vi "Write Listbox Data.vi"(8 "error in":errorcluster, 10 "Value":string[](array[string]), 11 "Listbox Ref in":refnum<vi>) -> (0 "error out":errorcluster, 3 "Listbox Ref out":refnum<vi>)   [LabVIEW 2020, in "G-Unicode.lvlib"]
uses:
  G-Unicode.lvlib
  Unicode/Controls/String Encoding.ctl
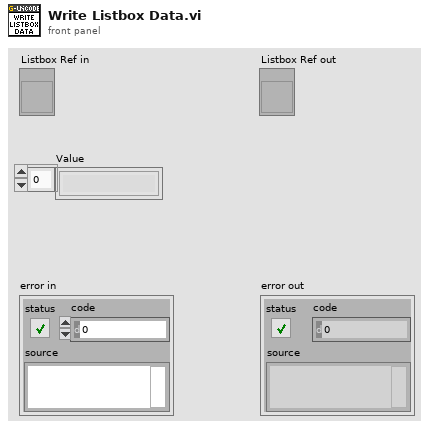
[diagram p1: front panel]
types:
  T1 = typedef "G-Unicode.lvlib/String Encoding.ctl" = enum16{"ANSI", "UTF-8", "UTF-16LE", "UTF-16BE", "Unknown"}
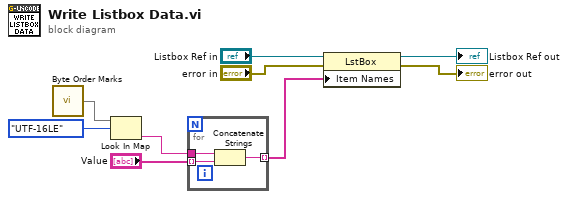
[diagram p0: block diagram]
diagram:
  n1 = call "Byte Order Marks.vi"() -> ("BOMs"=w5:map{T1, string})
  n2 = Look In Map(map=w5, key=String_Encoding."UTF-16LE") -> (value=w3:string)  [unwired: 1 in, 1 out]
  n3 = for {
    tunnel: "Value" -> [w12] mode=indexing
    tunnel: [w11] -> w1 mode=indexing
    tunnel: w3 -> [w10]
    n4 = Concatenate Strings(w10, w12) -> (w11:string)
  }
  n5 = property class="LstBox"(reference="Listbox Ref in", error in="error in", "Item Names"=w1) -> (reference out=→"Listbox Ref out":refnum<vi>, error out=→"error out":errorcluster)
